vi "Send Setup Pulse Waveform.vi"(5 "Spacing":dbl=50.0, 6 "Delay":dbl=50.0, 7 "Message Priority (Normal)":T2=enum."Normal", 8 "error in (no error)":errorcluster, 9 "Reset Pulse Conf":T1, 10 "Set Pulse Conf":T1, 11 "Message Enqueuer":refnum<class "Message Enqueuer.lvclass">) -> (0 "error out":errorcluster, 3 "Message Enqueuer out":refnum<class "Message Enqueuer.lvclass">)   [LabVIEW 2020, in "Actor_AFG.lvlib" / "Setup Pulse Waveform Msg.lvclass"]
doc: "This VI sends the message to an actor."
uses:
  Setup Pulse Waveform Msg.lvclass
  <vilib>/ActorFramework/Message Enqueuer/Message Enqueuer.lvclass
  <vilib>/ActorFramework/Message Enqueuer/Message Priority.ctl
  C:/Program Files/National Instruments/LabVIEW 2020/vi.lib/ActorFramework/Message/Message.lvclass
  Setup Pulse Waveform Msg.lvclass/Setup Pulse Waveform Msg.ctl
  <vilib>/ActorFramework/Message Enqueuer/Message Enqueuer.lvclass/Message Enqueuer.ctl
  <vilib>/ActorFramework/Message Priority Queue/Priority Enqueue.vi
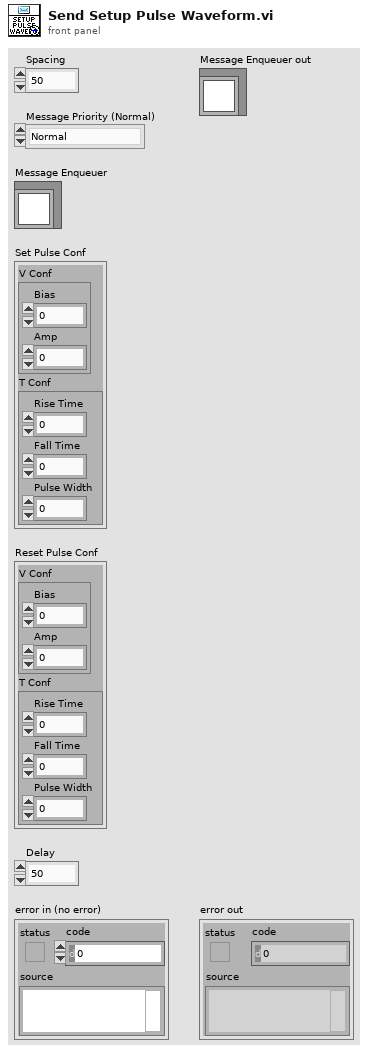
[diagram p1: front panel]
types:
  T1 = cluster{"V Conf":cluster{"Bias":dbl, "Amp":dbl}, "T Conf":cluster{"Rise Time":dbl, "Fall Time":dbl, "Pulse Width":dbl}}
  T2 = typedef "Actor Framework.lvlib/Message Enqueuer.lvclass/Message Priority.ctl" = enum16{"Low", "Normal", "High"}
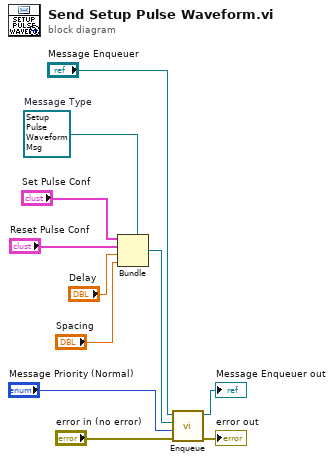
[diagram p0: block diagram]
diagram:
  w8 = refnum<class "Setup Pulse Waveform Msg.lvclass"> refnum  # Message Type
  n1 = Bundle(cluster=w8, "Set Pulse Conf", "Reset Pulse Conf", "Delay", "Spacing") -> (w7:refnum<class "Setup Pulse Waveform Msg.lvclass">)
  n2 = call <vilib>:"Enqueue.vi"("error in (no error)"="error in (no error)", "Message Priority (Normal)"="Message Priority (Normal)", "Message"=w7, "Message Enqueuer in"="Message Enqueuer") -> ("error out"=→"error out":errorcluster, "Message Enqueuer out"=→"Message Enqueuer out":refnum<class "Message Enqueuer.lvclass">)  [unwired: 6 in]
